vi "get dependency list.vi"(8 "error in":errorcluster, 11 "TBM Configuration Node in":refnum<class "TBM Configuration Node.lvclass">) -> (0 "error out":errorcluster, 2 "files":T1[](array[typedef]), 3 "TBM Configuration Node out":refnum<class "TBM Configuration Node.lvclass">)   [LabVIEW 2013, in "PL Framework Configuration Tool.lvlib" / "TBM Configuration Node.lvclass"]
uses:
  TBM Configuration Node.lvclass
  deployment configuration.ctl
  <vilib>/NI/Configuration Framework/Node/NISE_CEF_Node.lvclass/NISE_CEF_Node.ctl
  <vilib>/NI/Configuration Framework/Node/NISE_CEF_Node.lvclass
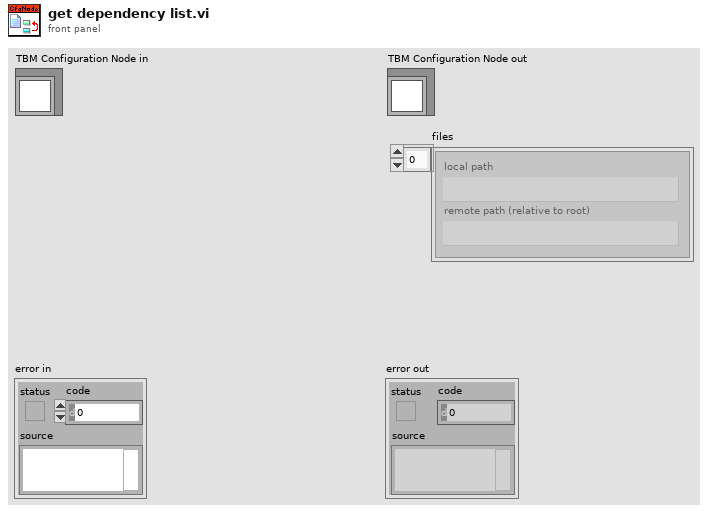
[diagram p1: front panel]
types:
  T1 = typedef "PL Framework Configuration Tool.lvlib/TBM Configuration Node.lvclass/deployment configuration.ctl" = cluster{"local path":path, "remote path (relative to root)":path}
  T2 = typedef "NISE_CEF_Node.lvclass/NodeRef.ctl" = refnum<data-value>
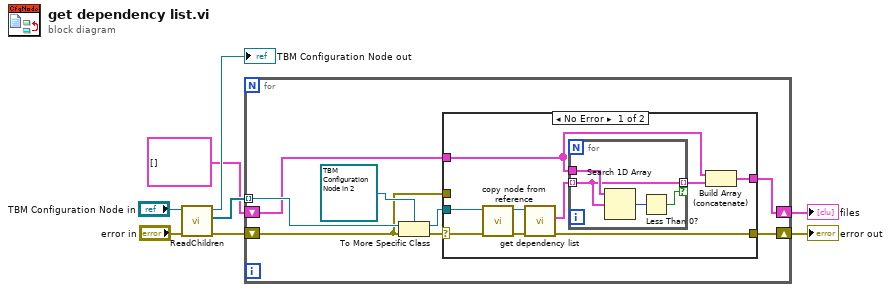
[diagram p0: block diagram]
diagram:
  n1 = call <vilib>:"ReadChildren.vi"("error in"="error in", "node in"="TBM Configuration Node in") -> ("error out"=w4:errorcluster, "output array"=w5:T2[], "node out"=→"TBM Configuration Node out":refnum<class "TBM Configuration Node.lvclass">)  [unwired: 7 in]
  n2 = for {
    tunnel: w5 -> [w16] mode=indexing
    shift-right: [w13] -> w3
    shift-left: w4 -> [w9]
    shift-right: [w10] -> w1
    shift-left: T1[] [] ("files") -> [w11]
    n3 = To More Specific Class(target class=refnum<data-value> refnum, reference=w16, error in=w9) -> (specific class reference=w12:refnum<data-value>, error out=w14:errorcluster)
    n4 = case shown="No Error" w14 {
      selector: w14 -> [w17 _]
      tunnel: [w22 w31] -> w13
      tunnel: w9 -> [_ w31]
      tunnel: w12 -> [w25 _]
      tunnel: w11 -> [w20 w30]
      tunnel: [w18 w30] -> w10
      frame No Error {
        n5 = call "copy node from reference.vi"("error in"=w17, "TBM node dvr"=w25) -> ("error out"=w23:errorcluster, "TBM node value"=w24:refnum<class "TBM Configuration Node.lvclass">)  [unwired: 8 in]
        n6 = call-dynamic "get dependency list.vi"("error in"=w23, "TBM Configuration Node in"=w24) -> ("error out"=w22:errorcluster, "files"=w21:T1[])  [unwired: 7 in, 1 out]
        n7 = for {
          tunnel: w21 -> [w27] mode=indexing
          tunnel: w20 -> [w29]
          tunnel: [w27] -> w19 mode=indexing if=w26
          n8 = Search 1D Array(1D array=w29, element=w27) -> (index of element=w28:i32)  [unwired: 1 in]
          n9 = Less Than 0?(x=w28) -> (x < 0?=w26:bool)
        }
        n10 = Build Array (concatenate)(w20, w19) -> (w18:T1[])
      }
      frame Error {
      }
    }
  }
  "error out" <- w3
  "files" <- w1
